vi "Flatten.vi"(8 "error in (no error)":errorcluster, 11 "Wavelength Digikröm in":refnum<class "Wavelength Digikröm.lvclass">) -> (0 "error out":errorcluster, 3 "Wavelength Digikröm out":refnum<class "Wavelength Digikröm.lvclass">)   [LabVIEW 2009, in "Wavelength Digikröm.lvclass"]
uses:
  Wavelength Digikröm.lvclass
  Scanner/Scanner.lvclass
  Wavelength Digikröm.lvclass/Wavelength Digikröm.ctl
  Global/File Locations.vi
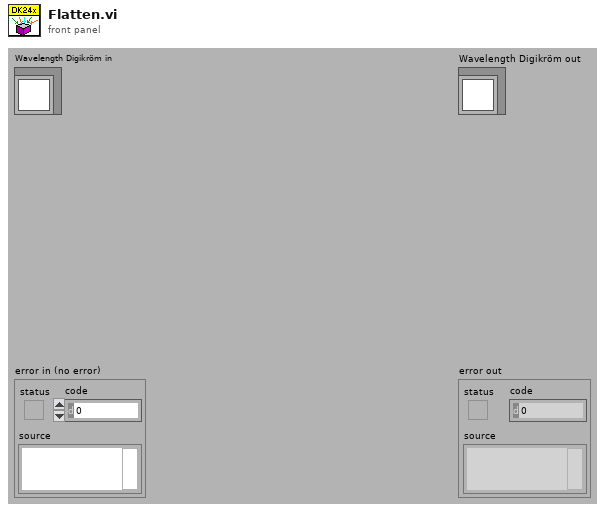
[diagram p1: front panel]
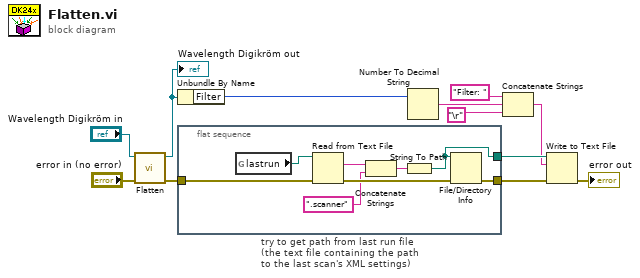
[diagram p0: block diagram]
diagram:
  n1 = call-parent "Flatten.vi"("error in (no error)"="error in (no error)", "Scanner in"="Wavelength Digikröm in") -> ("error out"=w10:errorcluster, "Scanner out"=w6:refnum<class "Wavelength Digikröm.lvclass">)  [unwired: 8 in]
  "Wavelength Digikröm out" <- w6
  n2 = Unbundle By Name(w6) -> ("Filter"=w5:u8)
  n3 = flat-sequence "try to get path from last run file\n(the text file containing the path\nto the last scan's XML settings)" {
    tunnel: [w20] -> w7
    tunnel: [w17] -> w8
    tunnel: w10 -> [w16]
    frame #0 {
      n4 = global read "File Locations.vi" "lastrun"() -> (w19:path)
      n5 = Read from Text File(file (use dialog)=w19, error in=w16) -> (text=w15:string, error out=w18:errorcluster)  [unwired: 4 out]
      n6 = Concatenate Strings(w15, ".scanner") -> (w13:string)
      n7 = String To Path(string=w13) -> (path=w20:path)
      n8 = File/Directory Info(path=w20, error in=w18) -> (error out=w17:errorcluster)  [unwired: 6 out]
    }
  }
  n9 = Number To Decimal String(number=w5) -> (decimal integer string=w3:string)  [unwired: 1 in]
  n10 = Concatenate Strings("Filter: ", w3, "\r") -> (w1:string)
  n11 = Write to Text File(file (use dialog)=w7, text=w1, error in=w8) -> (error out=→"error out":errorcluster)  [unwired: 1 in, 2 out]
